vi "L0_Maj_File_Appender.vi"(0 "Vin":dbl, 1 "CH":dbl, 2 "Att":dbl, 3 "IbClip":dbl=63.0, 4 "Clip":dbl=1.0, 5 "Vmeas":dbl, 6 "Threshold":dbl=1.0, 7 "file path (dialog if empty)":path, 9 "DT":dbl) -> ()   [LabVIEW 2012]
uses:
  <vilib>/Utility/file.llb/Write To Spreadsheet File (string).vi
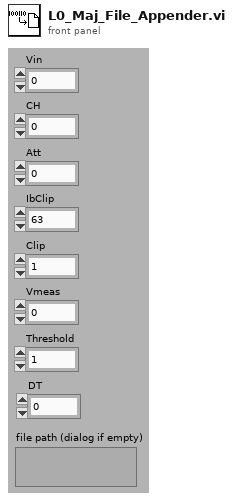
[diagram p1: front panel]
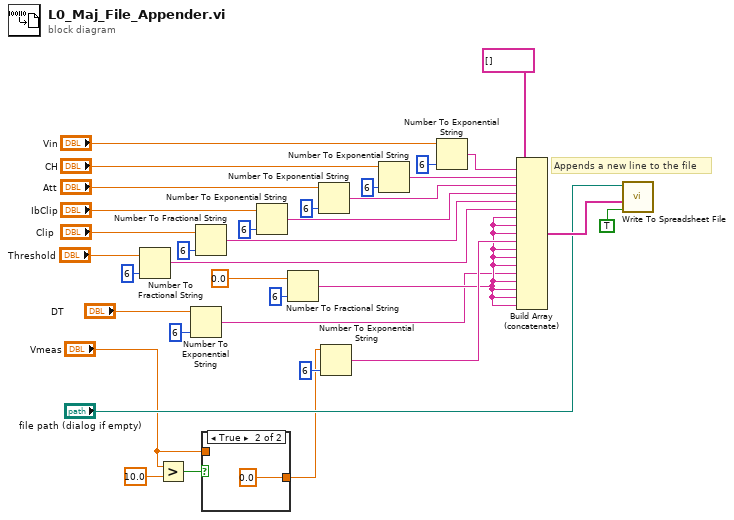
[diagram p0: block diagram]
diagram:
  # "Appends a new line to the file"
  n1 = Number To Fractional String(number="Threshold", precision (6)=i16 6) -> (F-format string=w11:string)  [unwired: 2 in]
  n2 = Greater?(x="Vmeas", y=10.0) -> (0:w3:bool)
  n3 = Number To Exponential String(number="DT", precision (6)=i16 6) -> (E-format string=w5:string)  [unwired: 2 in]
  n4 = Number To Fractional String(number="Clip", precision (6)=i16 6) -> (F-format string=w27:string)  [unwired: 2 in]
  n5 = case shown="True" w3 {
    tunnel: [w35 0.0 ("y")] -> w2
    tunnel: "Vmeas" -> [w35 _]
    frame False {
    }
    frame True {
    }
  }
  n6 = Number To Exponential String(number="IbClip", precision (6)=i16 6) -> (E-format string=w31:string)  [unwired: 2 in]
  n7 = Number To Fractional String(number=0.0, precision (6)=i16 6) -> (F-format string=w8:string)  [unwired: 2 in]
  n8 = Number To Exponential String(number="Att", precision (6)=i16 6) -> (E-format string=w33:string)  [unwired: 2 in]
  n9 = Number To Exponential String(number=w2, precision (6)=i16 6) -> (E-format string=w20:string)  [unwired: 2 in]
  n10 = Number To Exponential String(number="CH", precision (6)=i16 6) -> (E-format string=w34:string)  [unwired: 2 in]
  n11 = Number To Exponential String(number="Vin", precision (6)=i16 6) -> (E-format string=w26:string)  [unwired: 2 in]
  n12 = Build Array (concatenate)(string[] [] ("array"), w26, w34, w33, w31, w27, w11, w8, w8, w8, w20, w8, w8, w8, w5, w8, w8, w8, w8) -> (w22:string[])
  n13 = call-poly <vilib>:"Write To Spreadsheet File.vi"("append to file? (new file:F)"=TRUE, "1D data"=w22, "file path (dialog if empty)"="file path (dialog if empty)") -> ()  [unwired: 5 in, 1 out]
